vi "ShortcutMenu.vi"(8 "error in":errorcluster, 9 "menu ref in":refnum<k9>, 11 "node in":refnum<class "Page.lvclass">) -> (0 "error out":errorcluster, 1 "menu ref out":refnum<k9>, 3 "node out":refnum<class "Page.lvclass">)   [LabVIEW 2015, in "Page.lvclass"]
doc: "Defines the behavior of the shortcut menu of the node.Copyright 2015 National Instruments Corporation\n\nLicensed under the Apache License, Version 2.0 (the \"License\"); you may not use this file except in compliance with the License. You may obtain a copy of the License at http://www.apache.org/licenses/LICENSE-2.0\nUnless required by applicable law or agreed to in writing, software distributed under the License is distributed on an \"AS IS\" BASIS, WITHOUT WARRANTIES OR CONDITIONS OF ANY KIND, either express or implied. See the License for the specific language governing permissions and limitations under the License."
uses:
  Page.lvclass
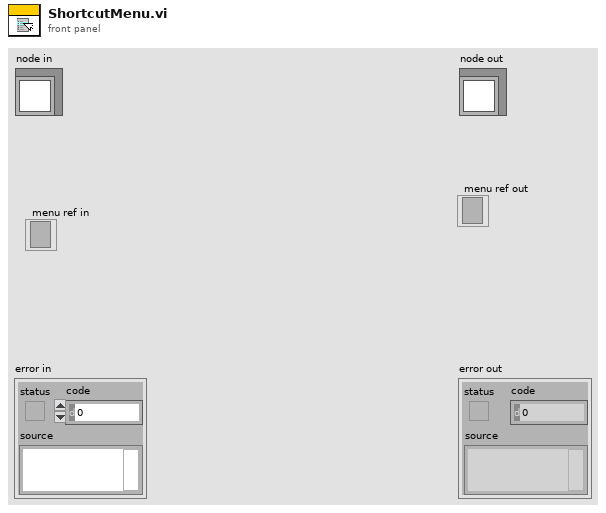
[diagram p1: front panel]
types:
  T1 = typedef "NISE_CEF_Node.lvclass/NodeMenuOptions.ctl" = cluster{"removable":bool, "movable":bool, "duplicate":bool}
  T2 = typedef "NISE_CEF_Node.lvclass/SubNodeCluster.ctl" = cluster{"subnodes menu name":string[], "subnodes class":string[]}
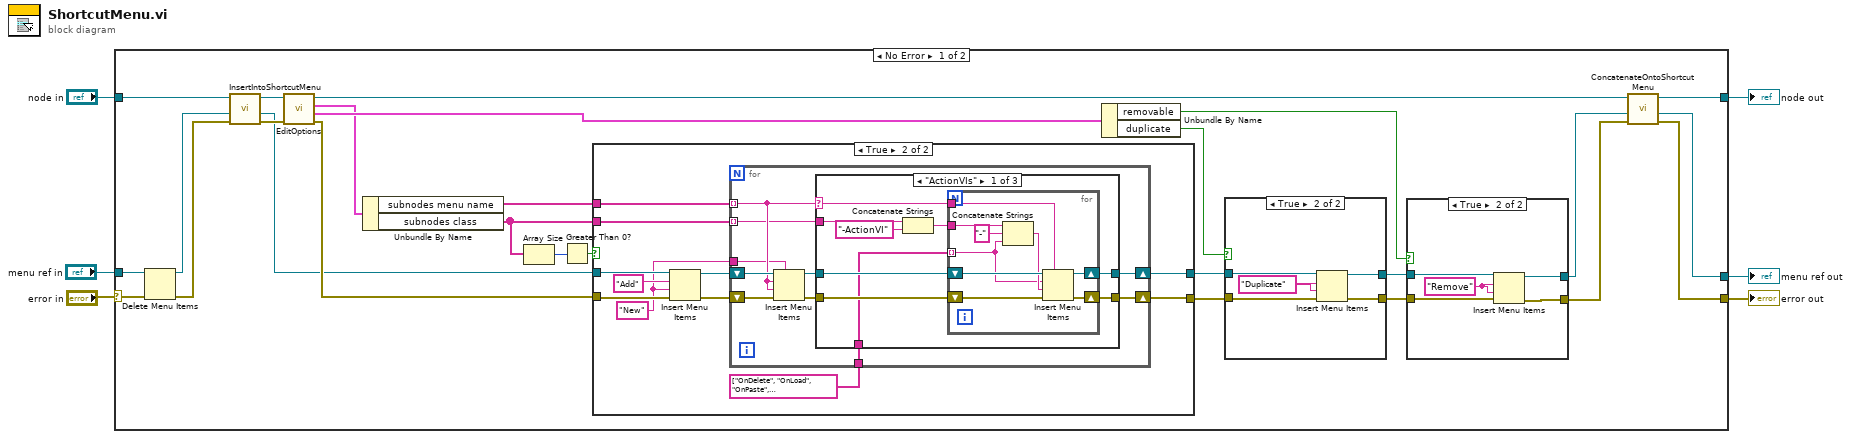
[diagram p0: block diagram]
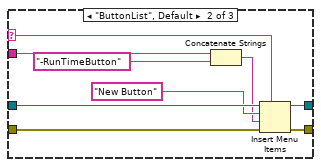
[diagram p5: hidden frame]
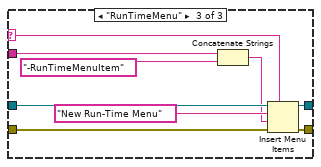
[diagram p6: hidden frame]
diagram:
  n1 = case shown="No Error" "error in" {
    selector: "error in" -> [w26 w108]
    tunnel: [w13 w109] -> w1
    tunnel: "node in" -> [w20 w109]
    tunnel: "menu ref in" -> [w29 w107]
    tunnel: [w11 w108] -> w3
    tunnel: [w9 w107] -> w2
    frame No Error {
      n2 = Delete Menu Items(6:w26, 9:w29) -> (0:w18:errorcluster, 3:w21:refnum<k9>)  [unwired: 2 in]
      n3 = call-dynamic "InsertIntoShortcutMenu.vi"("error in"=w18, "menu ref in"=w21, "node in"=w20) -> ("error out"=w17:errorcluster, "menu ref out"=w15:refnum<k9>, "node out"=w19:refnum<class "Page.lvclass">)  [unwired: 6 in]
      n4 = call-dynamic "EditOptions.vi"("error in"=w17, "node in"=w19) -> ("error out"=w16:errorcluster, "edit options"=w28:T1, "subnodes class"=w8:T2, "node out"=w14:refnum<class "Page.lvclass">)  [unwired: 6 in]
      n5 = Unbundle By Name(w8) -> ("subnodes menu name"=w22:string[], "subnodes class"=w7:string[])
      n6 = Array Size(array=w7) -> (size(s)=w33:i32)
      n7 = Greater Than 0?(x=w33) -> (x > 0?=w32:bool)
      n8 = case shown="True" w32 {
        tunnel: w15 -> [w49 w60]
        tunnel: w16 -> [w48 w59]
        tunnel: w22 -> [_ w56]
        tunnel: [w49 w55] -> w31
        tunnel: [w48 w54] -> w30
        tunnel: w7 -> [_ w52]
        frame False {
        }
        frame True {
          w51 = "New" ("item tags")
          n9 = Insert Menu Items(6:w59, 7:w51, 8:"Add", 9:w60) -> (0:w57:errorcluster, 3:w58:refnum<k9>)  [unwired: 2 in, 1 out]
          n10 = for {
            tunnel: w51 -> [w63]
            tunnel: w56 -> [w64] mode=indexing
            shift-right: [w70] -> w55
            shift-left: w58 -> [w68]
            shift-right: [w69] -> w54
            shift-left: w57 -> [w67]
            tunnel: w52 -> [w62] mode=indexing
            tunnel: string[] ["OnDelete", "OnLoad", "OnPaste", "OnTargetTypeChange", "OnDeleteRequest", "OnCompile", "OnSystemShutdown", "OnSave", "OnDownload"] ("Array") -> [w61]
            n11 = Insert Menu Items(5:w63, 6:w67, 7:w64, 8:w64, 9:w68) -> (0:w66:errorcluster, 3:w65:refnum<k9>)  [unwired: 1 in, 1 out]
            n12 = case shown="\"ActionVIs\"" w64 {
              selector: w64 -> [w75 w93 w102]
              tunnel: w65 -> [w79 w97 w106]
              tunnel: w66 -> [w78 w96 w105]
              tunnel: [w77 w95 w104] -> w70
              tunnel: [w76 w94 w103] -> w69
              tunnel: w62 -> [w73 w91 w99]
              tunnel: w61 -> [w71 _ _]
              frame "ActionVIs" {
                n13 = Concatenate Strings(w73, "-ActionVI" ("string")) -> (w72:string)
                n14 = for {
                  tunnel: w75 -> [w84]
                  shift-right: [w86] -> w77
                  shift-left: w79 -> [w88]
                  shift-right: [w85] -> w76
                  shift-left: w78 -> [w87]
                  tunnel: w72 -> [w83]
                  tunnel: w71 -> [w80] mode=indexing
                  n15 = Concatenate Strings(w83, "-" ("string"), w80) -> (w82:string)
                  n16 = Insert Menu Items(5:w84, 6:w87, 7:w82, 8:w80, 9:w88) -> (0:w85:errorcluster, 3:w86:refnum<k9>)  [unwired: 1 in, 1 out]
                }
              }
              frame "ButtonList", Default {
                n17 = Concatenate Strings(w91, "-RunTimeButton" ("string")) -> (w90:string)
                n18 = Insert Menu Items(5:w93, 6:w96, 7:w90, 8:"New Button" ("item names"), 9:w97) -> (0:w94:errorcluster, 3:w95:refnum<k9>)  [unwired: 1 in, 1 out]
              }
              frame "RunTimeMenu" {
                n19 = Concatenate Strings(w99, "-RunTimeMenuItem" ("string")) -> (w98:string)
                n20 = Insert Menu Items(5:w102, 6:w105, 7:w98, 8:"New Run-Time Menu" ("item names"), 9:w106) -> (0:w103:errorcluster, 3:w104:refnum<k9>)  [unwired: 1 in, 1 out]
              }
            }
          }
        }
      }
      n21 = Unbundle By Name(w28) -> ("removable"=w23:bool, "duplicate"=w27:bool)
      n22 = case shown="True" w27 {
        tunnel: w31 -> [w42 w47]
        tunnel: w30 -> [w41 w46]
        tunnel: [w42 w45] -> w24
        tunnel: [w41 w44] -> w25
        frame False {
        }
        frame True {
          w43 = "Duplicate"
          n23 = Insert Menu Items(6:w46, 7:w43, 8:w43, 9:w47) -> (0:w44:errorcluster, 3:w45:refnum<k9>)  [unwired: 2 in, 1 out]
        }
      }
      n24 = case shown="True" w23 {
        tunnel: w25 -> [w35 w40]
        tunnel: [w35 w39] -> w12
        tunnel: w24 -> [w34 w38]
        tunnel: [w34 w37] -> w10
        frame False {
        }
        frame True {
          w36 = "Remove"
          n25 = Insert Menu Items(6:w40, 7:w36, 8:w36, 9:w38) -> (0:w39:errorcluster, 3:w37:refnum<k9>)  [unwired: 2 in, 1 out]
        }
      }
      n26 = call-dynamic "ConcatenateOntoShortcutMenu.vi"("error in"=w12, "menu ref in"=w10, "node in"=w14) -> ("error out"=w11:errorcluster, "menu ref out"=w9:refnum<k9>, "node out"=w13:refnum<class "Page.lvclass">)  [unwired: 6 in]
    }
    frame Error {
    }
  }
  "error out" <- w3
  "node out" <- w1
  "menu ref out" <- w2
